vi "ReadConfig.vi"(8 "error in (no error)":errorcluster, 11 "GRMActor in":refnum<class "FlatFieldUI.lvclass">) -> (0 "error out":errorcluster, 3 "GRMActor out":refnum<class "FlatFieldUI.lvclass">)   [LabVIEW 2020, in "FlatFieldUI.lvlib" / "FlatFieldUI.lvclass"]
uses:
  FlatFieldUI.lvclass
  FlatFieldUI.lvclass/FlatFieldUI.ctl
  Hardware Abstraction Layer/Component/GenericActor/GenericActor/GenericController.lvclass
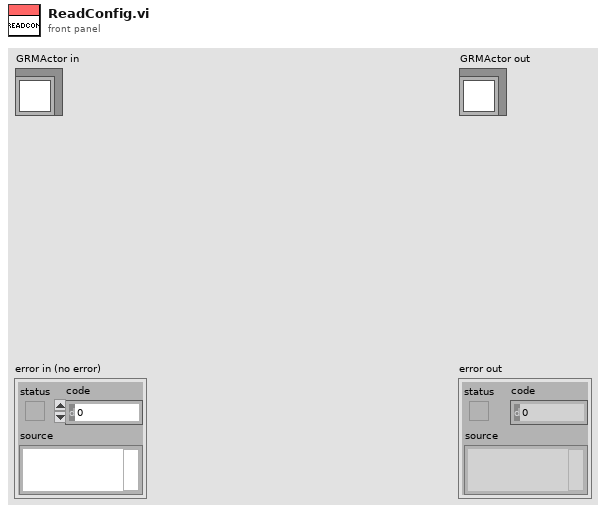
[diagram p1: front panel]
types:
  T1 = typedef "NI_LVConfig.lvlib/Config Data RefNum.ctl" = refnum<k1>
  T2 = cluster{"Values[0]":dbl, "Values[1]":dbl, "Values[2]":dbl}
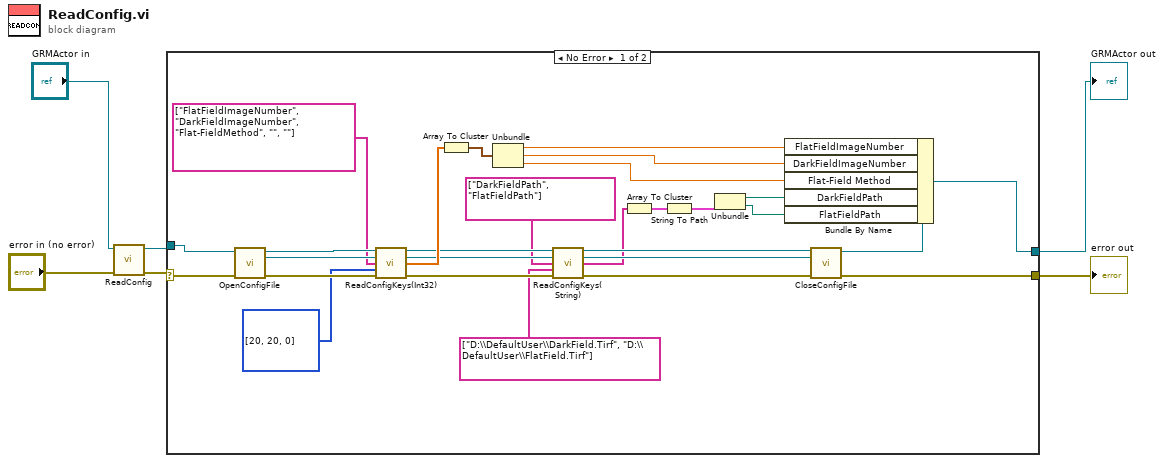
[diagram p0: block diagram]
diagram:
  n1 = call-parent "ReadConfig.vi"("error in (no error)"="error in (no error)", "GRMActor in"="GRMActor in") -> ("error out"=w3:errorcluster, "GRMActor out"=w4:refnum<class "FlatFieldUI.lvclass">)  [unwired: 8 in]
  n2 = case shown="No Error" w3 {
    selector: w3 -> [w34 w35]
    tunnel: [w26 w35] -> w1
    tunnel: [w29 w36] -> w2
    tunnel: w4 -> [w33 w36]
    frame No Error {
      n3 = call-dynamic "OpenConfigFile.vi"("error in (no error)"=w34, "GRMActor in"=w33) -> ("error out"=w32:errorcluster, "refnum"=w27:T1, "GRMActor out"=w30:refnum<class "FlatFieldUI.lvclass">)  [unwired: 7 in]
      n4 = call-dynamic "ReadConfigKeys(Int32).vi"("GRMActor in"=w30, "Config Refnum"=w27, "Keys"=string[] ["FlatFieldImageNumber", "DarkFieldImageNumber", "Flat-FieldMethod", "", ""] ("Values"), "Default"=i32[] [20, 20, 0], "error in (no error)"=w32) -> ("GRMActor out"=w17:refnum<class "FlatFieldUI.lvclass">, "Config Refnum dup"=w15:T1, "Values"=w24:dbl[], "error out"=w31:errorcluster)  [unwired: 7 in]
      n5 = Array To Cluster(array=w24) -> (cluster=w28:T2)
      n6 = Unbundle(w28) -> ("Values[0]"=w21:dbl, "Values[1]"=w20:dbl, "Values[2]"=w19:dbl)
      n7 = call-dynamic "ReadConfigKeys(String).vi"("GRMActor in"=w17, "Config Refnum"=w15, "Keys"=string[] ["DarkFieldPath", "FlatFieldPath"], "Values"=string[] ["D:\\DefaultUser\\DarkField.Tirf", "D:\\DefaultUser\\FlatField.Tirf"], "error in (no error)"=w31) -> ("GRMActor out"=w16:refnum<class "FlatFieldUI.lvclass">, "Config Refnum dup"=w14:T1, "Values"=w11:string[], "error out"=w18:errorcluster)  [unwired: 7 in]
      n8 = Array To Cluster(array=w11) -> (cluster=w10:cluster{"Values[0]":string, "Values[1]":string})
      n9 = String To Path(string=w10) -> (path=w9:cluster{"Values[0]":path, "Values[1]":path})
      n10 = Unbundle(w9) -> ("Values[0]"=w8:path, "Values[1]"=w7:path)
      n11 = call-dynamic "CloseConfigFile.vi"("error in (no error)"=w18, "refnum"=w14, "GRMActor in"=w16) -> ("error out"=w26:errorcluster, "GRMActor out"=w25:refnum<class "FlatFieldUI.lvclass">)  [unwired: 7 in]
      n12 = Bundle By Name(cluster=w25, "FlatFieldImageNumber"=w21, "DarkFieldImageNumber"=w20, "Flat-Field Method"=w19, "DarkFieldPath"=w8, "FlatFieldPath"=w7) -> (w29:refnum<class "FlatFieldUI.lvclass">)
    }
    frame Error {
    }
  }
  "error out" <- w1
  "GRMActor out" <- w2
